vi "Main.vi"(11 "Module Admin":refnum<class "Delacor_lib_QMH_Module Admin.lvclass">) -> ()   [LabVIEW 2025, in "Keyboard.lvlib"]
doc: "60% keyboard. 0-9, a-z (lowercase and uppercase), and all the standard symbols."
uses:
  Keyboard.lvlib
  <vilib>/Delacor/Delacor QMH/Libraries/Module Admin_class/Delacor_lib_QMH_Module Admin.lvclass
  Module Data--cluster.ctl
  <vilib>/Delacor/Delacor QMH/Libraries/Message Queue_class/Delacor_lib_QMH_Message Queue.lvclass/Delacor_lib_QMH_Message Queue.ctl
  Stop Argument--cluster.ctl
  <vilib>/Delacor/Delacor QMH/Libraries/Module Admin_class/Delacor_lib_QMH_Module Admin.lvclass/Delacor_lib_QMH_Module Admin.ctl
  Get VI Refnum Argument--cluster.ctl
  Get VI Refnum (Reply Payload)--cluster.ctl
  <vilib>/Utility/miscctls.llb/LVPointTypeDef.ctl
  <vilib>/Delacor/Delacor QMH/Libraries/Module Admin_class/Delacor_lib_QMH_Get External Launch.vi
  <vilib>/Delacor/Delacor QMH/Libraries/Message Queue_class/Delacor_lib_QMH_Enqueue Message (Single).vi
  <vilib>/Delacor/Delacor QMH/Libraries/Message Queue_class/Delacor_lib_QMH_Message Queue.lvclass
panel:
  in  "Clear Buffer":bool
  in  "Tab":bool
  in  "Space":bool
  in  "Send":bool
  in  "Output Type":bool
  out "Buffer":string
  in  "=+":bool
  in  "-_":bool
  in  "\\|":bool
  in  "]}":bool
  in  "[{":bool
  in  "'\"":bool
  in  ";:":bool
  in  "/?":bool
  in  ".>":bool
  in  ",<":bool
  in  "Enter":bool
  in  "Backspace":bool
  in  "0)":bool
  in  "9(":bool
  in  "8*":bool
  in  "7&":bool
  in  "6^":bool
  in  "5%":bool
  in  "4$":bool
  in  "3#":bool
  in  "2@":bool
  in  "1!":bool
  in  "Shift Right":bool
  in  "Caps":bool
  in  "Shift Left":bool
  in  "zZ":bool
  in  "yY":bool
  in  "xX":bool
  in  "wW":bool
  in  "vV":bool
  in  "uU":bool
  in  "tT":bool
  in  "sS":bool
  in  "rR":bool
  in  "qQ":bool
  in  "pP":bool
  in  "oO":bool
  in  "nN":bool
  in  "mM":bool
  in  "lL":bool
  in  "kK":bool
  in  "jJ":bool
  in  "iI":bool
  in  "hH":bool
  in  "gG":bool
  in  "fF":bool
  in  "eE":bool
  in  "dD":bool
  in  "cC":bool
  in  "bB":bool
  in  "aA":bool
  out "error out":errorcluster
  out "Status":string
  in  "Simulate MHL Error":bool
  in  "Simulate EHL Error":bool
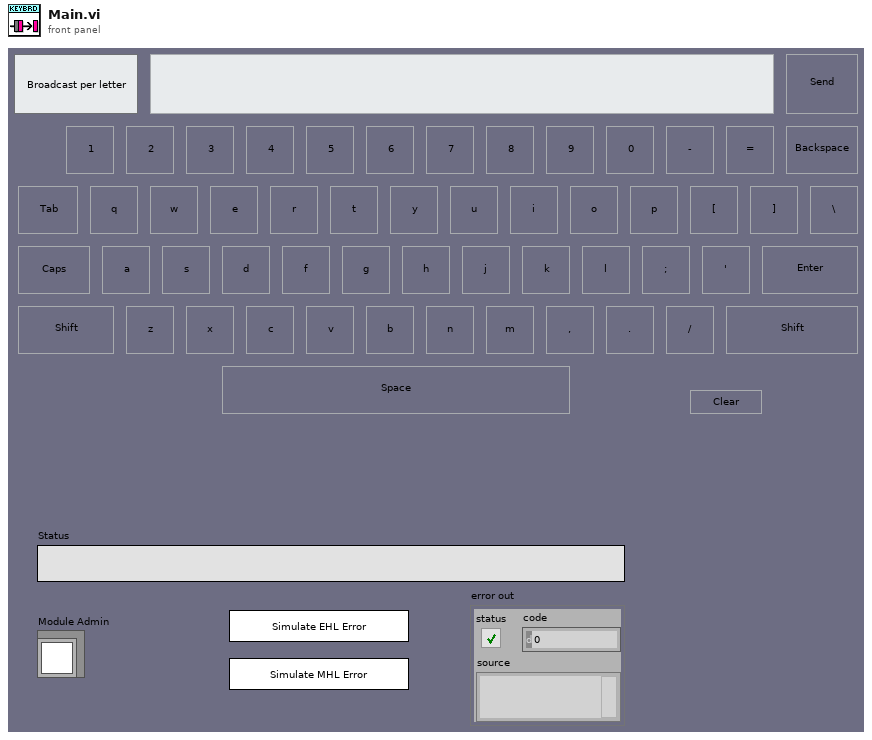
[diagram p1: front panel]
types:
  T1 = cluster{"=+":refnum<vi>, "-_":refnum<vi>, "\\|":refnum<vi>, "]}":refnum<vi>, "[{":refnum<vi>, "'\"":refnum<vi>, ";:":refnum<vi>, "/?":refnum<vi>, ".>":refnum<vi>, ",<":refnum<vi>, "0)":refnum<vi>, "9(":refnum<vi>, "8*":refnum<vi>, "7&":refnum<vi>, "6^":refnum<vi>, "5%":refnum<vi>, "4$":refnum<vi>, "3#":refnum<vi>, "2@":refnum<vi>, "1!":refnum<vi>, "eE":refnum<vi>, "rR":refnum<vi>, "cC":refnum<vi>, "kK":refnum<vi>, "yY":refnum<vi>, "fF":refnum<vi>, "gG":refnum<vi>, "hH":refnum<vi>, "mM":refnum<vi>, "zZ":refnum<vi>, "jJ":refnum<vi>, "uU":refnum<vi>, "tT":refnum<vi>, "sS":refnum<vi>, "wW":refnum<vi>, "xX":refnum<vi>, "iI":refnum<vi>, "qQ":refnum<vi>, "dD":refnum<vi>, "lL":refnum<vi>, "vV":refnum<vi>, "pP":refnum<vi>, "oO":refnum<vi>, "nN":refnum<vi>, "bB":refnum<vi>, "aA":refnum<vi>}
  T2 = typedef "Keyboard.lvlib/Request Events--cluster.ctl" = cluster{"Stop Module":refnum<user-event>, "Show Panel":refnum<user-event>, "Hide Panel":refnum<user-event>, "Get Module Execution Status":refnum<user-event>, "Show Diagram":refnum<user-event>, "Get VI Refnum":refnum<user-event>}
  T3 = typedef "Keyboard.lvlib/Module Data--cluster.ctl" = cluster{"Buffer":string, "Shift Status":bool}
  T4 = enum8{"Enabled", "Disabled", "Disabled and Grayed Out"}
  T5 = enum32{"invalid lock state", "Not Locked", "Locked (No Password)", "Password-protected"}
  T6 = typedef "Keyboard.lvlib/Stop Argument--cluster.ctl" = cluster{"Origin":string, "Exit via Stop Module Req?":bool, "Wait for Module to stop?":bool}
  T7 = typedef "Keyboard.lvlib/Get VI Refnum Argument--cluster.ctl" = cluster{"Wait Notifier":refnum<notifier>, "wait for reply":bool}
  T8 = typedef "LVPointTypeDef.ctl" = cluster{"Horizontal":i16, "Vertical":i16}
  T9 = enum32{"Invalid", "Standard", "Closed", "Hidden", "Minimized", "Maximized"}
  T10 = typedef "Keyboard.lvlib/Get VI Refnum (Reply Payload)--cluster.ctl" = cluster{"VI Refnum":refnum<vi>, "error":errorcluster}
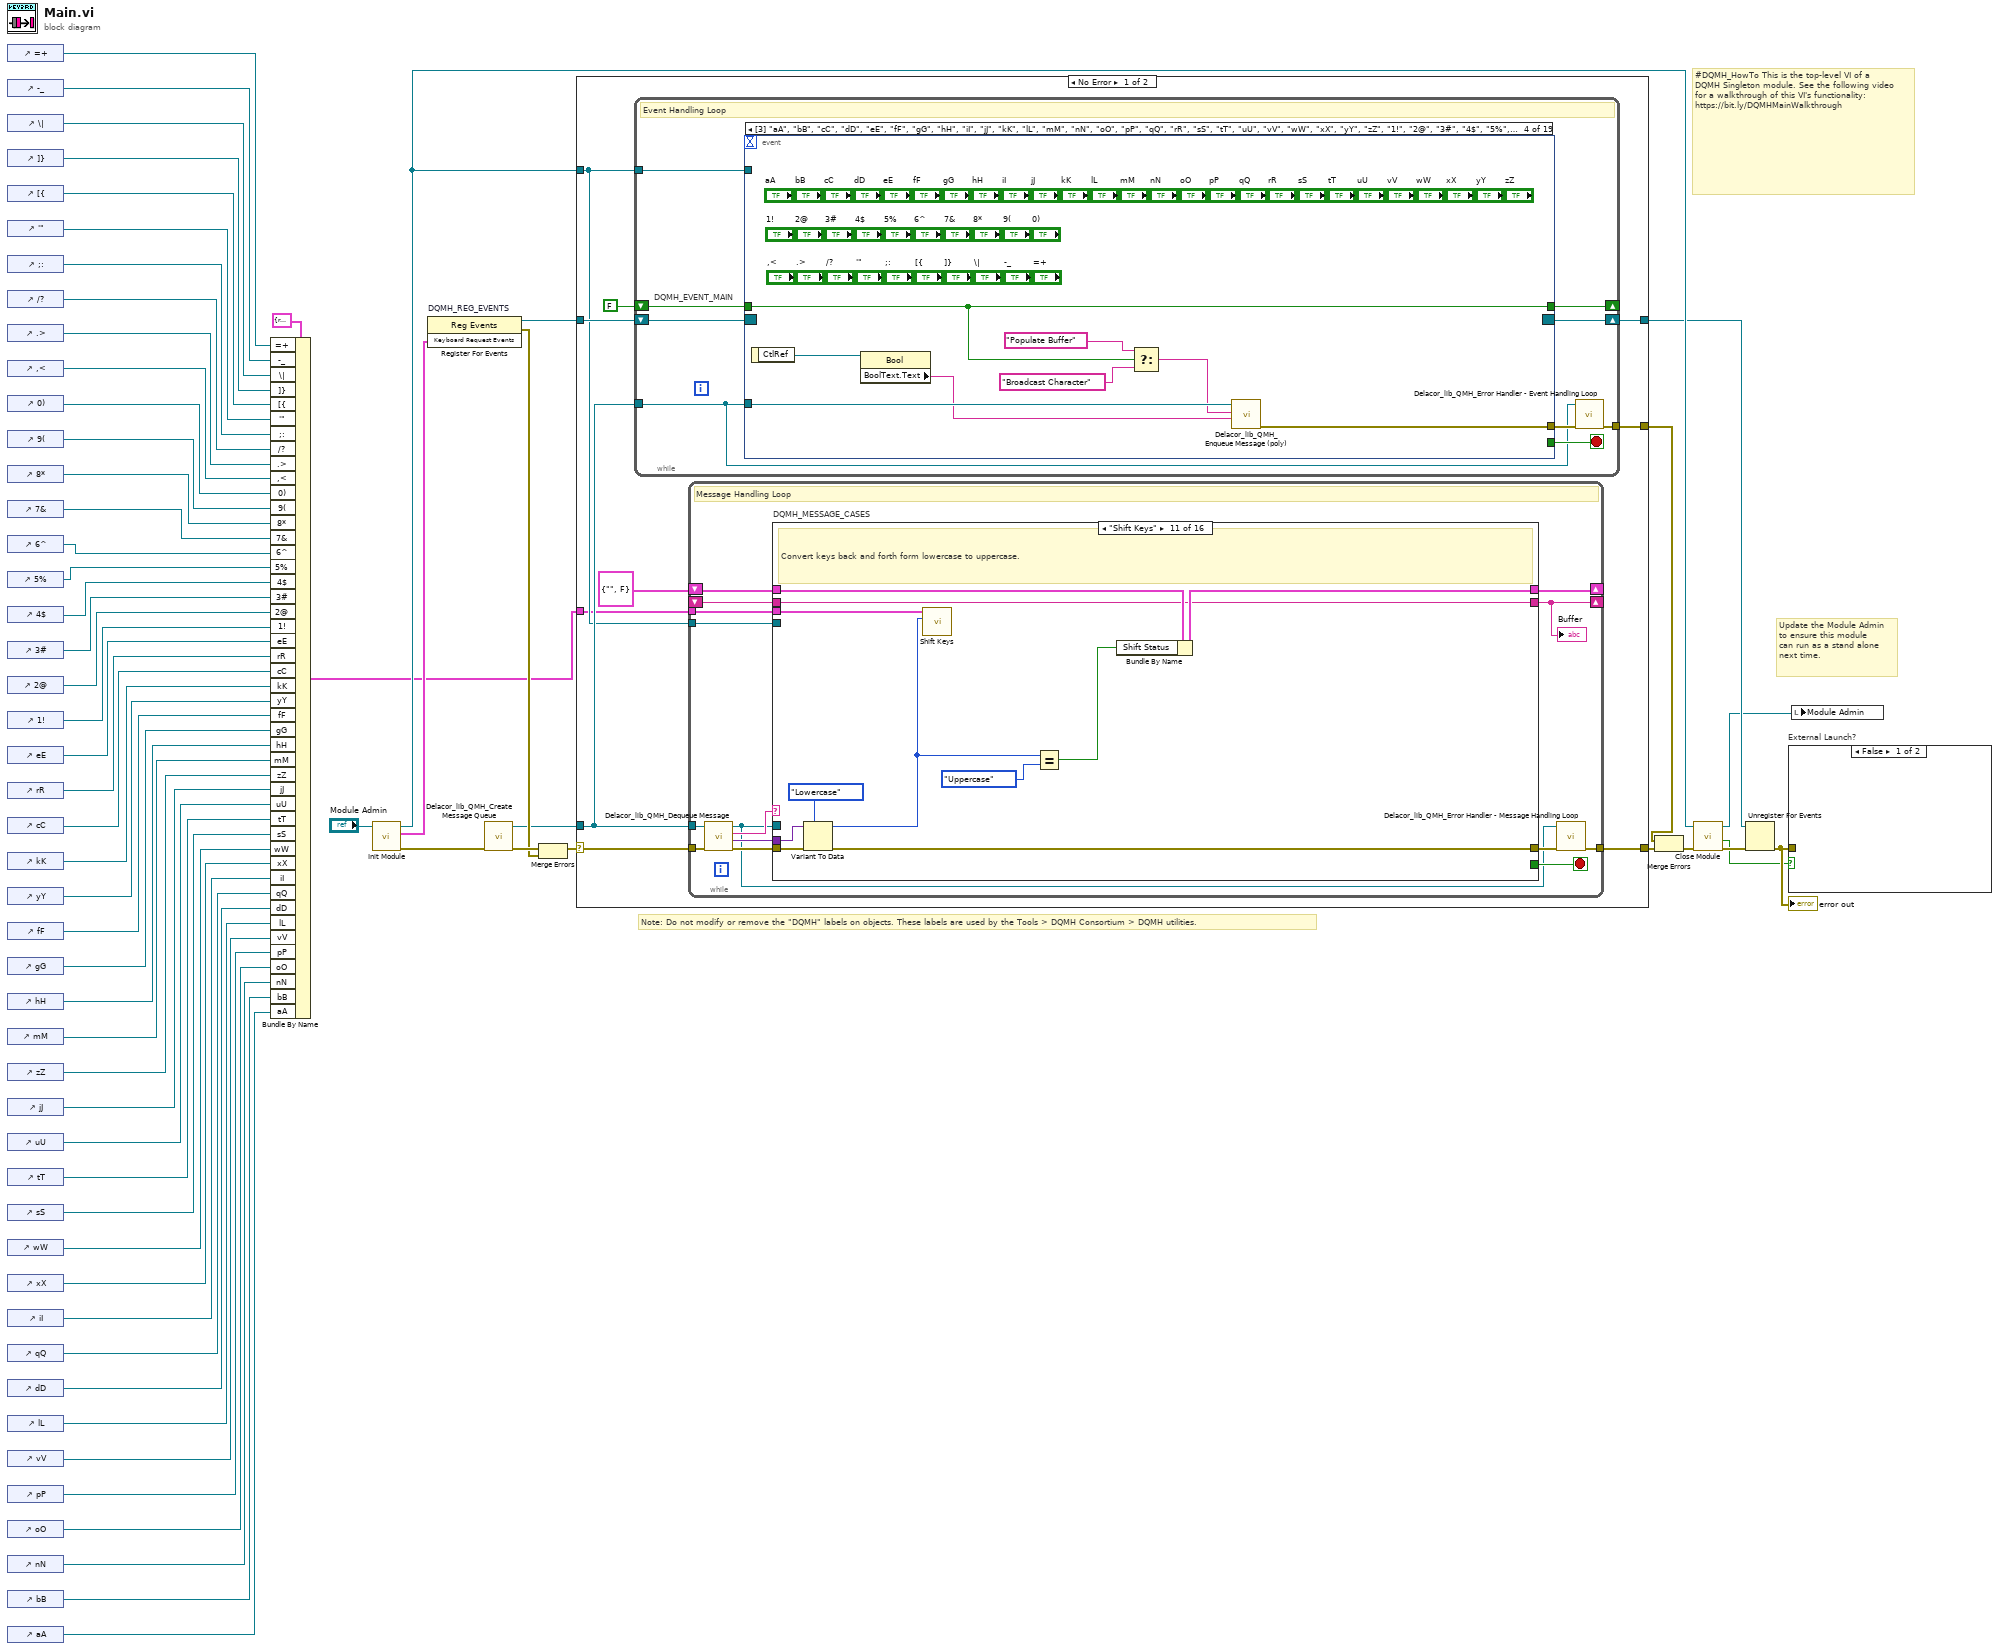
[diagram p0: block diagram]
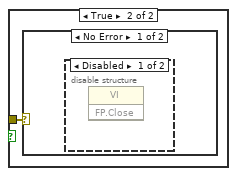
[diagram p2: hidden frame]
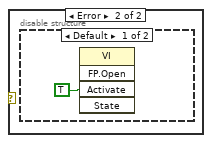
[diagram p4: hidden frame]
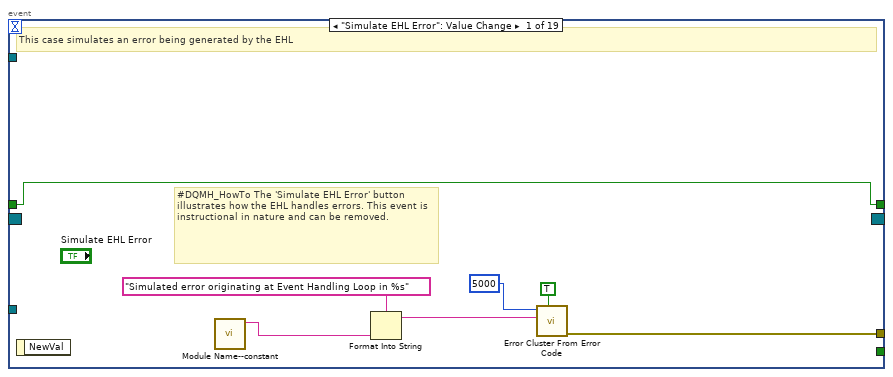
[diagram p6: hidden frame]
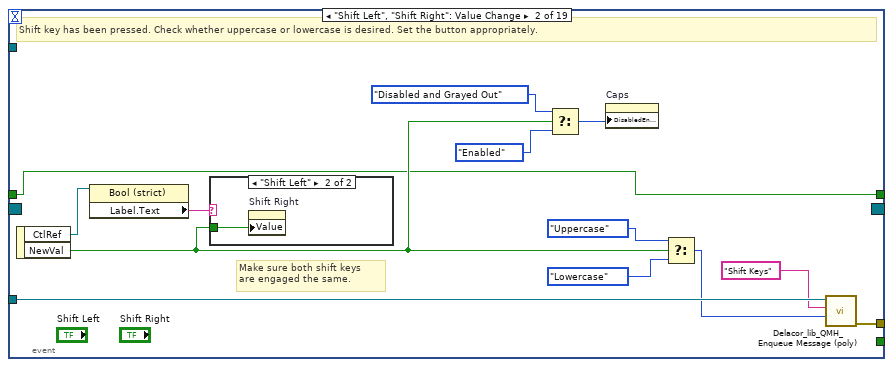
[diagram p7: hidden frame]
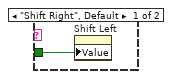
[diagram p8: hidden frame]
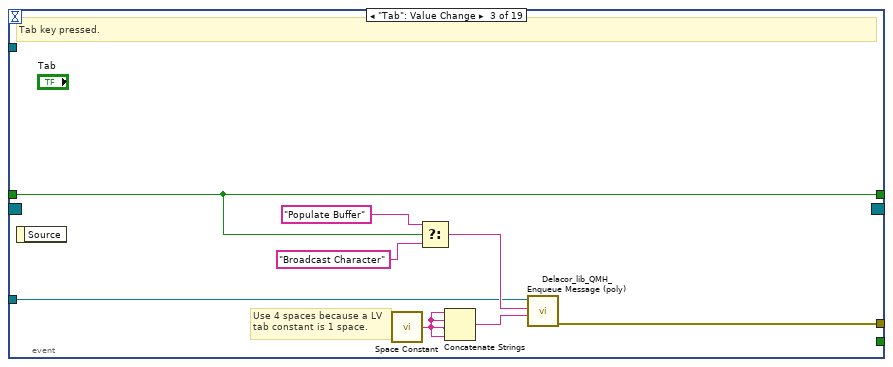
[diagram p9: hidden frame]
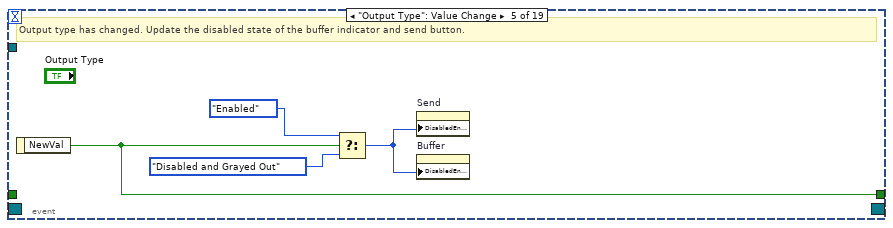
[diagram p10: hidden frame]
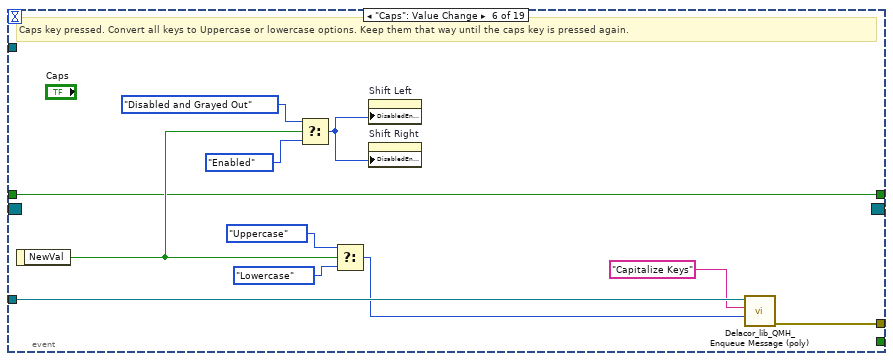
[diagram p11: hidden frame]
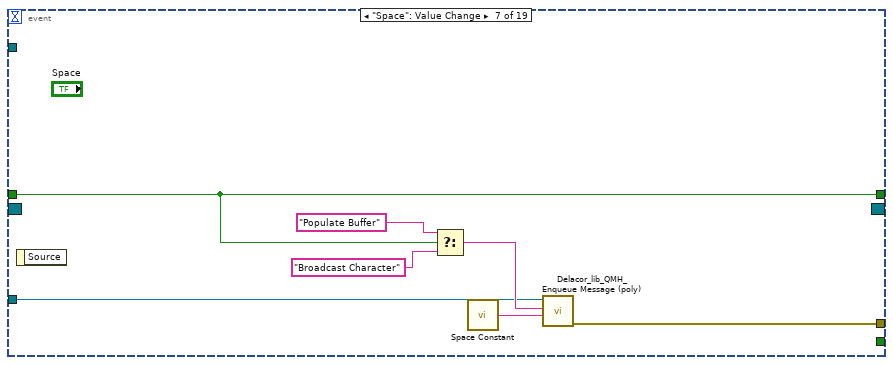
[diagram p12: hidden frame]
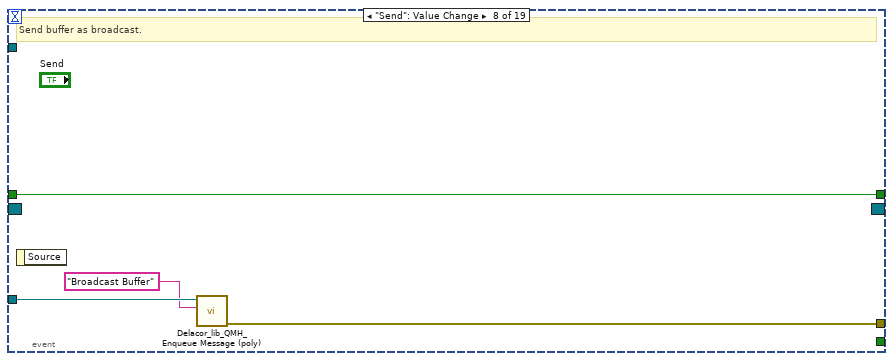
[diagram p13: hidden frame]
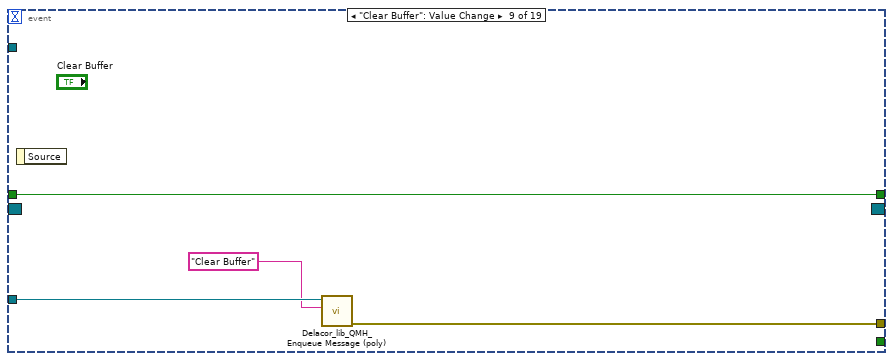
[diagram p14: hidden frame]
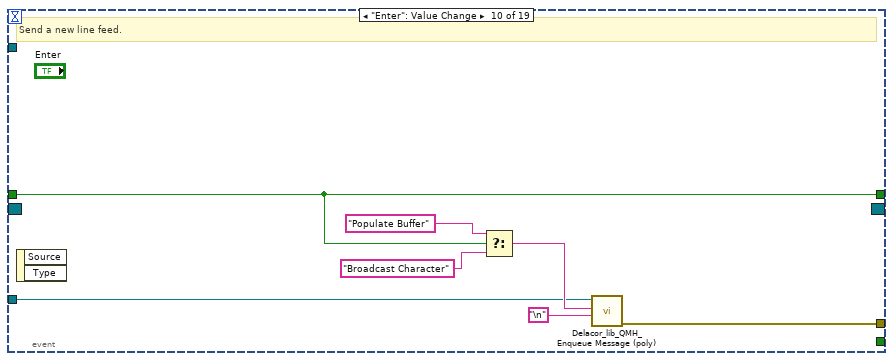
[diagram p15: hidden frame]
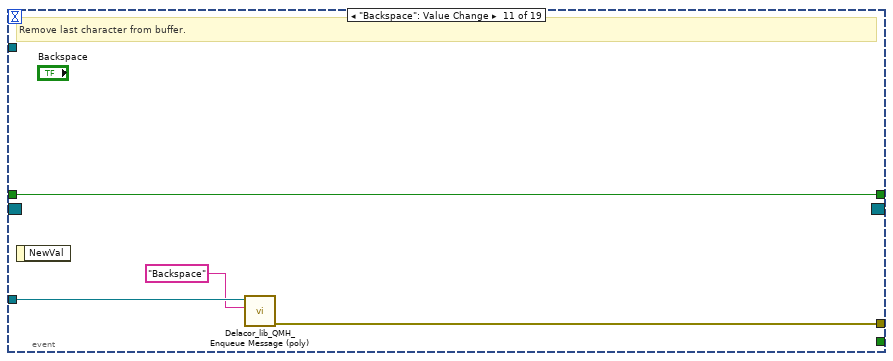
[diagram p16: hidden frame]
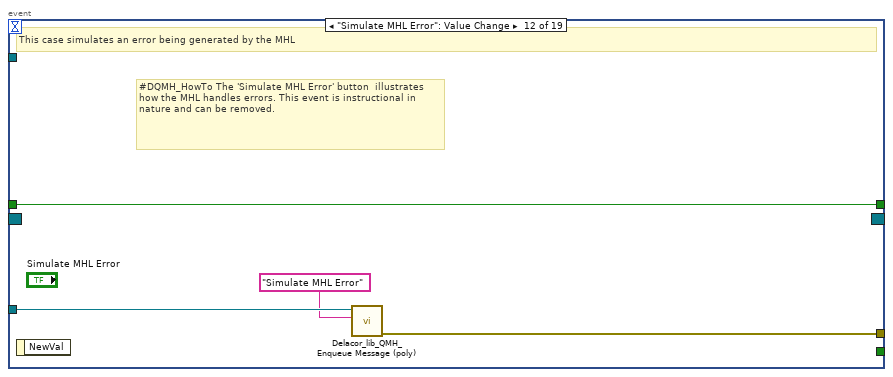
[diagram p17: hidden frame]
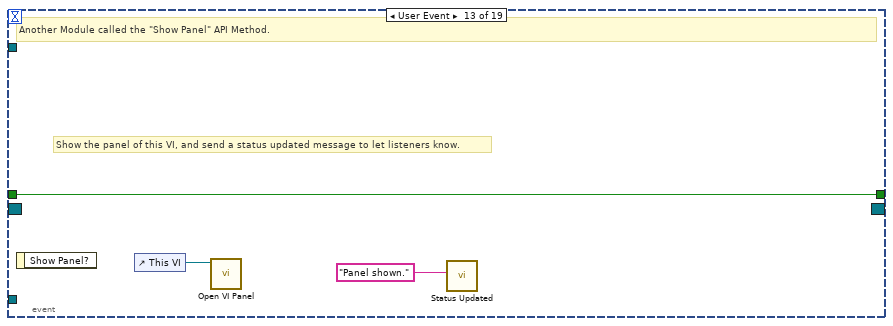
[diagram p18: hidden frame]
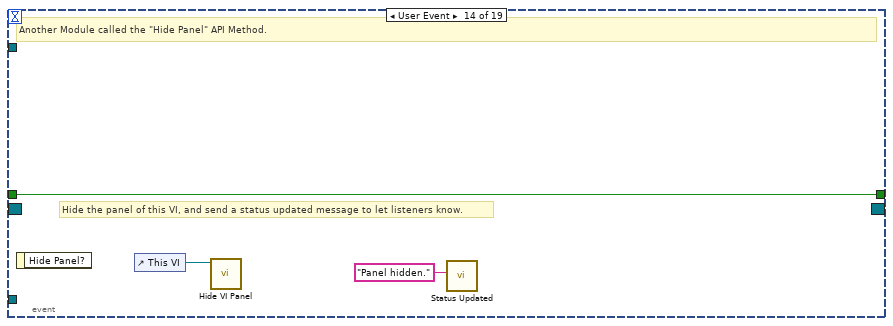
[diagram p19: hidden frame]
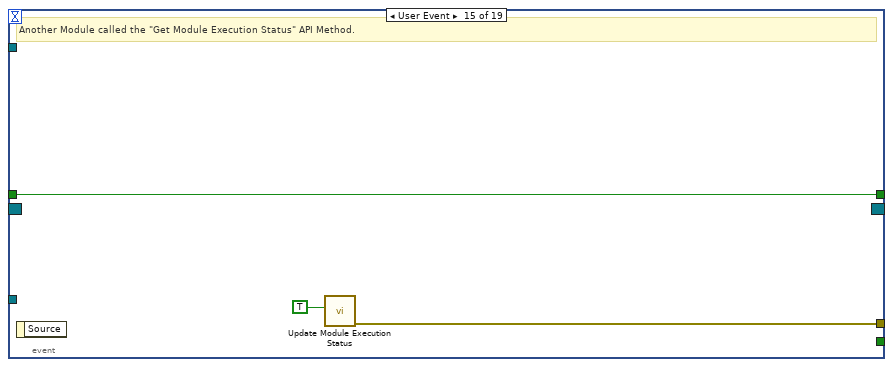
[diagram p20: hidden frame]
diagram:
  # "#DQMH_HowTo This is the top-level VI of a DQMH Singleton module. See the following video for a walkthrough of this VI's functionality: https://bit.ly/DQMHMainWalkthrough"
  # "Note: Do not modify or remove the \"DQMH\" labels on objects. These labels are used by the Tools > DQMH Consortium > DQMH utilities."
  # "Update the Module Admin to ensure this module can run as a stand alone next time."
  n1 = control-ref of="=+"() -> (w48:refnum<vi>)
  n2 = control-ref of="-_"() -> (w47:refnum<vi>)
  n3 = control-ref of="\\|"() -> (w46:refnum<vi>)
  n4 = control-ref of="]}"() -> (w45:refnum<vi>)
  n5 = control-ref of="[{"() -> (w44:refnum<vi>)
  n6 = control-ref of="'\""() -> (w43:refnum<vi>)
  n7 = control-ref of=";:"() -> (w42:refnum<vi>)
  n8 = control-ref of="/?"() -> (w41:refnum<vi>)
  n9 = control-ref of=".>"() -> (w40:refnum<vi>)
  n10 = control-ref of=",<"() -> (w39:refnum<vi>)
  n11 = control-ref of="0)"() -> (w38:refnum<vi>)
  n12 = control-ref of="9("() -> (w37:refnum<vi>)
  n13 = control-ref of="8*"() -> (w36:refnum<vi>)
  n14 = control-ref of="7&"() -> (w35:refnum<vi>)
  n15 = control-ref of="6^"() -> (w34:refnum<vi>)
  n16 = control-ref of="5%"() -> (w33:refnum<vi>)
  n17 = control-ref of="4$"() -> (w32:refnum<vi>)
  n18 = control-ref of="3#"() -> (w31:refnum<vi>)
  n19 = control-ref of="2@"() -> (w30:refnum<vi>)
  n20 = control-ref of="1!"() -> (w29:refnum<vi>)
  n21 = control-ref of="eE"() -> (w28:refnum<vi>)
  n22 = control-ref of="rR"() -> (w27:refnum<vi>)
  n23 = control-ref of="cC"() -> (w26:refnum<vi>)
  n24 = control-ref of="kK"() -> (w25:refnum<vi>)
  n25 = control-ref of="yY"() -> (w24:refnum<vi>)
  n26 = control-ref of="fF"() -> (w23:refnum<vi>)
  n27 = control-ref of="gG"() -> (w22:refnum<vi>)
  n28 = control-ref of="hH"() -> (w21:refnum<vi>)
  n29 = control-ref of="mM"() -> (w20:refnum<vi>)
  n30 = control-ref of="zZ"() -> (w19:refnum<vi>)
  n31 = control-ref of="jJ"() -> (w18:refnum<vi>)
  n32 = control-ref of="uU"() -> (w17:refnum<vi>)
  n33 = control-ref of="tT"() -> (w16:refnum<vi>)
  n34 = control-ref of="sS"() -> (w15:refnum<vi>)
  n35 = control-ref of="wW"() -> (w14:refnum<vi>)
  n36 = control-ref of="xX"() -> (w13:refnum<vi>)
  n37 = control-ref of="iI"() -> (w12:refnum<vi>)
  n38 = control-ref of="qQ"() -> (w11:refnum<vi>)
  n39 = control-ref of="dD"() -> (w10:refnum<vi>)
  n40 = control-ref of="lL"() -> (w9:refnum<vi>)
  n41 = control-ref of="vV"() -> (w8:refnum<vi>)
  n42 = control-ref of="pP"() -> (w7:refnum<vi>)
  n43 = control-ref of="oO"() -> (w6:refnum<vi>)
  n44 = control-ref of="nN"() -> (w5:refnum<vi>)
  n45 = control-ref of="bB"() -> (w4:refnum<vi>)
  n46 = control-ref of="aA"() -> (w3:refnum<vi>)
  n47 = Bundle By Name(cluster=T1 {"=+"=refnum, "-_"=refnum, "\\|"=refnum, "]}"=refnum, "[{"=refnum, "'\""=refnum, ";:"=refnum, "/?"=refnum, ".>"=refnum, ",<"=refnum, "0)"=refnum, "9("=refnum, "8*"=refnum, "7&"=refnum, "6^"=refnum, "5%"=refnum, "4$"=refnum, "3#"=refnum, "2@"=refnum, "1!"=refnum, "eE"=refnum, "rR"=refnum, "cC"=refnum, "kK"=refnum, "yY"=refnum, "fF"=refnum, "gG"=refnum, "hH"=refnum, "mM"=refnum, "zZ"=refnum, "jJ"=refnum, "uU"=refnum, "tT"=refnum, "sS"=refnum, "wW"=refnum, "xX"=refnum, "iI"=refnum, "qQ"=refnum, "dD"=refnum, "lL"=refnum, "vV"=refnum, "pP"=refnum, "oO"=refnum, "nN"=refnum, "bB"=refnum, "aA"=refnum}, "=+"=w48, "-_"=w47, "\\|"=w46, "]}"=w45, "[{"=w44, "'\""=w43, ";:"=w42, "/?"=w41, ".>"=w40, ",<"=w39, "0)"=w38, "9("=w37, "8*"=w36, "7&"=w35, "6^"=w34, "5%"=w33, "4$"=w32, "3#"=w31, "2@"=w30, "1!"=w29, "eE"=w28, "rR"=w27, "cC"=w26, "kK"=w25, "yY"=w24, "fF"=w23, "gG"=w22, "hH"=w21, "mM"=w20, "zZ"=w19, "jJ"=w18, "uU"=w17, "tT"=w16, "sS"=w15, "wW"=w14, "xX"=w13, "iI"=w12, "qQ"=w11, "dD"=w10, "lL"=w9, "vV"=w8, "pP"=w7, "oO"=w6, "nN"=w5, "bB"=w4, "aA"=w3) -> (w1:T1)
  n48 = call "Init Module.vi"("Singleton Module Admin in"="Module Admin") -> ("error out"=w64:errorcluster, "Keyboard Request Events"=w53:T2, "Singleton Module Admin out"=w56:refnum<class "Delacor_lib_QMH_Module Admin.lvclass">)  [unwired: 8 in]
  n49 = register-events "DQMH_REG_EVENTS"(w53) -> (reference out=w54:refnum<event-registration>, error out=w57:errorcluster)  [unwired: 2 in]
  n50 = call <vilib>:"Delacor_lib_QMH_Create Message Queue.vi"("error in"=w64) -> ("error out"=w59:errorcluster, "Message Queue"=w52:refnum<class "Delacor_lib_QMH_Message Queue.lvclass">)  [unwired: 9 in]
  n51 = Merge Errors(w59, w57) -> (w58:errorcluster)
  n52 = case shown="No Error" w58 {
    selector: w58 -> [w73 w406]
    tunnel: [w75 w405] -> w65
    tunnel: [w72 w404] -> w55
    tunnel: w54 -> [w70 w404]
    tunnel: w52 -> [w69 w399]
    tunnel: [w74 _] -> w62
    tunnel: w56 -> [w68 w400]
    tunnel: w1 -> [w67 _]
    frame No Error {
      n53 = while {
        tunnel: w69 -> [w78]
        shift-right: [w81] -> w72
        shift-left: w70 -> [w82]
        tunnel: [w83] -> w74
        tunnel: w68 -> [w79]
        shift-right: [w77] -> _
        shift-left: FALSE ("NewVal") -> [w76]
        stop <- w80 stop-if-true
        # "Event Handling Loop"
        n54 = event "DQMH_EVENT_MAIN" shown="[3] \"aA\", \"bB\", \"cC\", \"dD\", \"eE\", \"fF\", \"gG\", \"hH\", \"iI\", \"jJ\", \"kK\", \"lL\", \"mM\", \"nN\", \"oO\", \"pP\", \"qQ\", \"rR\", \"sS\", \"tT\", \"uU\", \"vV\", \"wW\", \"xX\", \"yY\", \"zZ\", \"1!\", \"2@\", \"3#\", \"4$\", \"5%\", \"6^\", \"7&\", \"8*\", \"9(\", \"0)\", \",<\", \".>\", \"/?\", \";:\", \"'\"\", \"[{\", \"]}\", \"\\|\", \"-_\", \"=+\": Value Change" {
          selector: w82 -> [_ _ _ _ _ _ _ _ _ _ _ _ _ _ _ _ _ _ _]
          dyn-events: [_ _ _ _ _ _ _ _ _ _ _ _ _ _ _ _ _ _ _] -> w81
          timeout: _ -> [_ _ _ _ _ _ _ _ _ _ _ _ _ _ _ _ _ _ _]
          tunnel: [_ _ _ _ _ _ _ _ _ _ _ _ _ _ _ _ TRUE ("Discard?") _ _] -> w80
          tunnel: w78 -> [_ w104 w110 w121 _ w137 w141 w148 w152 w154 w163 w166 _ _ _ _ w195 w203 w219]
          tunnel: [w91 w103 w109 w120 _ w136 w140 w147 w151 w153 w162 w167 _ _ w176 _ w198 w205 w213] -> w84
          tunnel: w79 -> [_ _ _ _ _ _ _ _ _ _ _ _ _ _ _ _ _ w202 _]
          tunnel: [w85 w92 w107 w115 w123 w127 w139 w145 w149 w156 w160 w164 w168 w171 w174 w177 w187 w200 w220] -> w77
          tunnel: w76 -> [w85 w92 w107 w115 _ w127 w139 w145 w149 w156 w160 w164 w168 w171 w174 w177 w187 w200 w220]
          event "Simulate EHL Error": Value Change {
            # "#DQMH_HowTo The 'Simulate EHL Error' button  illustrates how the EHL handles errors. This event is instructional in nature and can be removed."
            # "This case simulates an error being generated by the EHL"
            n55 = event-data() -> ()  [unwired: 1 in, 1 out]
            n56 = call "Module Name--constant.vi"() -> ("Module Name"=w88:string)  [unwired: 11 in]
            n57 = Format Into String(format string="Simulated error originating at Event Handling Loop in %s", w88) -> (resulting string=w89:string)  [unwired: 2 in, 1 out]
            n58 = call <vilib>:"Error Cluster From Error Code.vi"("show call chain? (False)"=TRUE, "error message (\"\")"=w89, "error code (0)"=5000) -> ("error out"=w91:errorcluster)  [unwired: 6 in]
          }
          event "Shift Left", "Shift Right": Value Change {
            # "Make sure both shift keys\nare engaged the same."
            # "Shift key has been pressed. Check whether uppercase or lowercase is desired. Set the button appropriately."
            n59 = event-data() -> ("CtlRef"=w98:refnum<vi>, "NewVal"=w94:bool)  [unwired: 1 in]
            n60 = property class="Bool (strict)"(reference=w98) -> ("Label.Text"=w97:string)  [unwired: 1 in, 2 out]
            n61 = case shown="\"Shift Left\"" w97 {
              tunnel: w94 -> [w105 w106]
              frame "Shift Right", Default {
                n62 = property on="Shift Left" class="Bool (strict)"("Value"=w105) -> ()  [unwired: 2 in, 2 out]
              }
              frame "Shift Left" {
                n63 = property on="Shift Right" class="Bool (strict)"("Value"=w106) -> ()  [unwired: 2 in, 2 out]
              }
            }
            n64 = Select(t=T4."Disabled and Grayed Out" ("Disabled"), s=w94, f=T4."Enabled" ("Disabled")) -> (s? t:f=w93:T4)
            n65 = property on="Caps" class="Bool (strict)"("DisabledEnum"=w93) -> ()  [unwired: 2 in, 2 out]
            n66 = Select(t=enum16{"Uppercase", "Lowercase"}."Uppercase" ("Upper / Lower Case"), s=w94, f=enum16{"Uppercase", "Lowercase"}."Lowercase" ("Upper / Lower Case")) -> (s? t:f=w99:enum16{"Uppercase", "Lowercase"})
            n67 = call-poly <vilib>:"Delacor_lib_QMH_Enqueue Message (poly).vi"("Message Data"=w99, "Message"="Shift Keys", "Message Queue in"=w104) -> ("error out"=w103:errorcluster)  [unwired: 7 in, 1 out]
          }
          event "Tab": Value Change {
            # "Use 4 spaces because a LV\ntab constant is 1 space."
            # "Tab key pressed."
            n68 = event-data() -> ()  [unwired: 1 in, 1 out]
            n69 = call <vilib>:"Space Constant.vi"() -> ("String"=w114:string)
            n70 = Select(t="Populate Buffer", s=w107, f="Broadcast Character" ("t")) -> (s? t:f=w113:string)
            n71 = Concatenate Strings(w114, w114, w114, w114) -> (w108:string)
            n72 = call-poly <vilib>:"Delacor_lib_QMH_Enqueue Message (poly).vi"("Message Data"=w108, "Message"=w113, "Message Queue in"=w110) -> ("error out"=w109:errorcluster)  [unwired: 7 in, 1 out]
          }
          event "aA", "bB", "cC", "dD", "eE", "fF", "gG", "hH", "iI", "jJ", "kK", "lL", "mM", "nN", "oO", "pP", "qQ", "rR", "sS", "tT", "uU", "vV", "wW", "xX", "yY", "zZ", "1!", "2@", "3#", "4$", "5%", "6^", "7&", "8*", "9(", "0)", ",<", ".>", "/?", ";:", "'\"", "[{", "]}", "\\|", "-_", "=+": Value Change {
            n73 = event-data() -> ("CtlRef"=w122:refnum<vi>)  [unwired: 1 in]
            n74 = property class="Bool"(reference=w122) -> ("BoolText.Text"=w118:string)  [unwired: 1 in, 2 out]
            n75 = Select(t="Populate Buffer", s=w115, f="Broadcast Character" ("t")) -> (s? t:f=w119:string)
            n76 = call-poly <vilib>:"Delacor_lib_QMH_Enqueue Message (poly).vi"("Message Data"=w118, "Message"=w119, "Message Queue in"=w121) -> ("error out"=w120:errorcluster)  [unwired: 7 in, 1 out]
          }
          event "Output Type": Value Change {
            # "Output type has changed. Update the disabled state of the buffer indicator and send button."
            n77 = event-data() -> ("NewVal"=w123:bool)  [unwired: 1 in]
            n78 = Select(t=T4."Enabled" ("Disabled"), s=w123, f=T4."Disabled and Grayed Out" ("Disabled")) -> (s? t:f=w125:T4)
            n79 = property on="Send" class="Bool"("DisabledEnum"=w125) -> ()  [unwired: 2 in, 2 out]
            n80 = property on="Buffer" class="Str"("DisabledEnum"=w125) -> ()  [unwired: 2 in, 2 out]
          }
          event "Caps": Value Change {
            # "Caps key pressed. Convert all keys to Uppercase or lowercase options. Keep them that way until the caps key is pressed again."
            n81 = event-data() -> ("NewVal"=w131:bool)  [unwired: 1 in]
            n82 = Select(t=T4."Disabled and Grayed Out" ("Disabled"), s=w131, f=T4."Enabled" ("Disabled")) -> (s? t:f=w128:T4)
            n83 = Select(t=enum16{"Uppercase", "Lowercase"}."Uppercase" ("Upper / Lower Case"), s=w131, f=enum16{"Uppercase", "Lowercase"}."Lowercase" ("Upper / Lower Case")) -> (s? t:f=w132:enum16{"Uppercase", "Lowercase"})
            n84 = property on="Shift Left" class="Bool (strict)"("DisabledEnum"=w128) -> ()  [unwired: 2 in, 2 out]
            n85 = property on="Shift Right" class="Bool (strict)"("DisabledEnum"=w128) -> ()  [unwired: 2 in, 2 out]
            n86 = call-poly <vilib>:"Delacor_lib_QMH_Enqueue Message (poly).vi"("Message Data"=w132, "Message"="Capitalize Keys", "Message Queue in"=w137) -> ("error out"=w136:errorcluster)  [unwired: 7 in, 1 out]
          }
          event "Space": Value Change {
            n87 = event-data() -> ()  [unwired: 1 in, 1 out]
            n88 = Select(t="Populate Buffer", s=w139, f="Broadcast Character" ("t")) -> (s? t:f=w144:string)
            n89 = call <vilib>:"Space Constant.vi"() -> ("String"=w138:string)
            n90 = call-poly <vilib>:"Delacor_lib_QMH_Enqueue Message (poly).vi"("Message Data"=w138, "Message"=w144, "Message Queue in"=w141) -> ("error out"=w140:errorcluster)  [unwired: 7 in, 1 out]
          }
          event "Send": Value Change {
            # "Send buffer as broadcast."
            n91 = event-data() -> ()  [unwired: 1 in, 1 out]
            n92 = call-poly <vilib>:"Delacor_lib_QMH_Enqueue Message (poly).vi"("Message"="Broadcast Buffer", "Message Queue in"=w148) -> ("error out"=w147:errorcluster)  [unwired: 8 in, 1 out]
          }
          event "Clear Buffer": Value Change {
            n93 = event-data() -> ()  [unwired: 1 in, 1 out]
            n94 = call-poly <vilib>:"Delacor_lib_QMH_Enqueue Message (poly).vi"("Message"="Clear Buffer", "Message Queue in"=w152) -> ("error out"=w151:errorcluster)  [unwired: 8 in, 1 out]
          }
          event "Enter": Value Change {
            # "Send a new line feed."
            n95 = event-data() -> ()  [unwired: 1 in, 2 out]
            n96 = Select(t="Populate Buffer", s=w156, f="Broadcast Character" ("t")) -> (s? t:f=w159:string)
            n97 = call-poly <vilib>:"Delacor_lib_QMH_Enqueue Message (poly).vi"("Message Data"="\n", "Message"=w159, "Message Queue in"=w154) -> ("error out"=w153:errorcluster)  [unwired: 7 in, 1 out]
          }
          event "Backspace": Value Change {
            # "Remove last character from buffer."
            n98 = event-data() -> ()  [unwired: 1 in, 1 out]
            n99 = call-poly <vilib>:"Delacor_lib_QMH_Enqueue Message (poly).vi"("Message"="Backspace", "Message Queue in"=w163) -> ("error out"=w162:errorcluster)  [unwired: 8 in, 1 out]
          }
          event "Simulate MHL Error": Value Change {
            # "#DQMH_HowTo The 'Simulate MHL Error' button  illustrates how the MHL handles errors. This event is instructional in nature and can be removed."
            # "This case simulates an error being generated by the MHL"
            n100 = event-data() -> ()  [unwired: 1 in, 1 out]
            n101 = call-poly <vilib>:"Delacor_lib_QMH_Enqueue Message (poly).vi"("Message"="Simulate MHL Error", "Message Queue in"=w166) -> ("error out"=w167:errorcluster)  [unwired: 8 in, 1 out]
          }
          event User Event {
            # "Show the panel of this VI, and send a status updated message to let listeners know."
            # "Another Module called the \"Show Panel\" API Method."
            n102 = event-data() -> ()  [unwired: 1 in, 1 out]
            n103 = control-ref of="This VI"() -> (w170:refnum<vi>)
            n104 = call "Open VI Panel.vi"("VI"=w170) -> ()  [unwired: 10 in, 1 out]
            n105 = call "Status Updated.vi"("Status"="Panel shown." ("format string")) -> ()  [unwired: 10 in, 1 out]
          }
          event User Event {
            # "Hide the panel of this VI, and send a status updated message to let listeners know."
            # "Another Module called the \"Hide Panel\" API Method."
            n106 = event-data() -> ()  [unwired: 1 in, 1 out]
            n107 = control-ref of="This VI"() -> (w173:refnum<vi>)
            n108 = call "Hide VI Panel.vi"("VI"=w173) -> ()  [unwired: 10 in, 1 out]
            n109 = call "Status Updated.vi"("Status"="Panel hidden." ("format string")) -> ()  [unwired: 10 in, 1 out]
          }
          event User Event {
            # "Another Module called the \"Get Module Execution Status\" API Method."
            n110 = event-data() -> ()  [unwired: 1 in, 1 out]
            n111 = call "Update Module Execution Status.vi"("Running?"=TRUE) -> ("error out"=w176:errorcluster)  [unwired: 10 in]
          }
          event User Event {
            # "Another Module called the \"Show Diagram\" API Method. This event is used for debugging."
            n112 = event-data() -> ()  [unwired: 1 in, 1 out]
            n113 = disable-structure shown="RUN_TIME_ENGINE==False" {
              frame condition #0 (active) {
                # "functionality not available in exe"
                n114 = invoke on="Invoke Node" class="VI" method="Lock State.Get"() -> (error out=w183:errorcluster, "Get Lock State"=w182:T5, "pwd in cache"=w179:bool)  [unwired: 4 in, 1 out]
                n115 = Equal?(x=T5."Password-protected", y=w182) -> (x = y?=w180:bool)
                n116 = Compound Arithmetic op=AND(w180, invert w179) -> (w178:bool)
                n117 = case shown="False" w178 {
                  tunnel: w183 -> [w186 _]
                  frame False {
                    n118 = property on="Property Node" class="VI"(error in=w186, "BDWin.Open"=TRUE ("Block Diagram Window:Open")) -> ()  [unwired: 1 in, 2 out]
                    n119 = call "Status Updated.vi"("Status"="Block Diagram shown." ("format string")) -> ()  [unwired: 10 in, 1 out]
                  }
                  frame True {
                    # "Password-protected VI, and the password is not in the cache. Do not show the diagram."
                  }
                }
              }
              frame condition #1 {
              }
            }
          }
          event User Event {
            # "The Stop Module Event can get fired from the Exit message in the MHL. The queue gets destroyed in that case. If the queue no longer exists, the Enqueue Exit as a priority message will return error 1. It is safe to ignore, because the module is already exiting."
            # "Another Module called the \"Stop Module\" API Method  or the Message Handling Loop below."
            n120 = event-data() -> ("Origin"=w194:string, "Exit via Stop Module Req?"=w190:bool, "Wait for Module to stop?"=w189:bool)  [unwired: 1 in]
            n121 = local write "Status"(w194) -> ()
            n122 = Bundle By Name(cluster=T6 {"Origin"="", "Exit via Stop Module Req?"=FALSE, "Wait for Module to stop?"=FALSE} ("Stop Argument"), "Exit via Stop Module Req?"=w190, "Wait for Module to stop?"=w189) -> (w188:T6)
            n123 = call-poly <vilib>:"Delacor_lib_QMH_Enqueue Message (poly).vi"("Priority Message? (F)"=TRUE, "Message Data"=w188, "Message"="Exit", "Message Queue in"=w195) -> ("error out"=w199:errorcluster)  [unwired: 6 in, 1 out]
            n124 = call <vilib>:"Clear Errors.vi"("error in (no error)"=w199, "specific error code to clear (0: all)"=1) -> ("error out"=w198:errorcluster)  [unwired: 4 in, 1 out]
          }
          event Panel Close? {
            w204 = TRUE  # Discard the event, the MHL is responsible for closing and stopping this VI.
            # "Hide the panel or send the 'Exit' message if the user clicks the 'X' on the module main VI panel."
            n125 = event-data() -> ()  [unwired: 1 in, 1 out]
            n126 = property on="Property Node" class="Module Admin"(reference=w202) -> ("Accessors:External Launch"=w201:bool)  [unwired: 1 in, 2 out]
            n127 = case shown="False" w201 {
              tunnel: w203 -> [_ w211]
              tunnel: [_ w212] -> w205
              frame True {
                # "If externally launched, clicking the 'X' hides the panel, but doesn't close it."
                n128 = control-ref of="This VI"() -> (w208:refnum<vi>)
                n129 = call "Hide VI Panel.vi"("VI"=w208) -> ("error out"=w206:errorcluster)  [unwired: 10 in]
                n130 = call "Status Updated.vi"("error in"=w206, "Status"="Panel hidden." ("format string")) -> ()  [unwired: 9 in, 1 out]
              }
              frame False {
                # "If run as a stand-alone VI, clicking the panel 'X' stops the VI."
                n131 = call-poly <vilib>:"Delacor_lib_QMH_Enqueue Message (poly).vi"("Priority Message? (F)"=TRUE, "Message"="Exit", "Message Queue in"=w211) -> ("error out"=w212:errorcluster)  [unwired: 7 in, 1 out]
              }
            }
            n132 = event-data ("Event Filter Node")("Discard?"=w204) -> ()  [unwired: 1 in, 1 out]
          }
          event User Event {
            # "Another Module called the \"Get VI Refnum\" API Method."
            n133 = event-data() -> ("Wait Notifier"=w215:refnum<notifier>, "wait for reply"=w214:bool)  [unwired: 1 in]
            n134 = Bundle(cluster=T7 {"Wait Notifier"=refnum, "wait for reply"=FALSE} ("Get VI Refnum Argument"), "Wait Notifier"=w215, "wait for reply"=w214) -> (w216:T7)
            n135 = call-poly <vilib>:"Delacor_lib_QMH_Enqueue Message (poly).vi"("Message Data"=w216, "Message"="Get VI Refnum", "Message Queue in"=w219) -> ("error out"=w213:errorcluster)  [unwired: 7 in, 1 out]
          }
        }
        n136 = call-dynamic "Delacor_lib_QMH_Error Handler - Event Handling Loop.vi"("error in"=w84, "Message Queue in"=w78) -> ("dup error in"=w83:errorcluster)  [unwired: 8 in, 1 out]
      }
      n137 = while {
        tunnel: w69 -> [w224]
        shift-right: [w232] -> _
        shift-left: T3 {"Buffer"="", "Shift Status"=FALSE} ("Data Cluster") -> [w233]
        tunnel: w73 -> [w235]
        tunnel: [w227] -> w75
        tunnel: w68 -> [w228]
        tunnel: w67 -> [w223]
        shift-right: [w222] -> _
        shift-left: _ -> [w221]
        stop <- w231 stop-if-true
        # "Message Handling Loop"
        n138 = call-dynamic "Delacor_lib_QMH_Dequeue Message.vi"("error in"=w235, "Message Queue in"=w224) -> ("error out"=w234:errorcluster, "Message Data"=w229:variant, "Message"=w230:string, "Message Queue out"=w225:refnum<class "Delacor_lib_QMH_Message Queue.lvclass">)  [unwired: 6 in]
        n139 = case "DQMH_MESSAGE_CASES" shown="\"Shift Keys\"" w230 {
          selector: w230 -> [_ _ _ _ _ _ _ _ _ _ _ _ _ _ _ w394]
          tunnel: w225 -> [_ _ _ _ _ _ _ _ _ _ _ _ _ w358 w381 _]
          tunnel: w234 -> [w257 w262 w275 w281 w285 w290 w294 w307 w317 w329 w340 w343 w353 w365 w387 w397]
          tunnel: [w255 w262 w264 w280 w285 w288 w294 w303 w316 w326 w337 w343 w352 w361 w382 w398] -> w226
          tunnel: w233 -> [w246 w261 w274 w279 w284 w287 w293 w300 w313 w328 w339 w342 w350 w360 w380 w395]
          tunnel: [w245 w261 w274 w279 w283 w287 w292 w300 w311 w328 w332 w342 w350 w360 w380 w395] -> w232
          tunnel: [_ _ _ _ _ _ _ _ _ _ _ _ _ _ w379 _] -> w231
          tunnel: w229 -> [_ _ w271 _ _ _ _ w306 w315 w325 w336 _ _ w359 w378 _]
          tunnel: w228 -> [w247 _ _ _ _ _ _ _ _ _ _ _ _ w357 w373 _]
          tunnel: w223 -> [_ _ _ _ _ _ _ _ _ w327 w338 _ _ _ _ _]
          tunnel: [w237 w260 w273 w278 w282 w289 w291 w301 w309 w322 w330 w341 w344 w354 w372 w388] -> w222
          tunnel: w221 -> [_ w260 w273 w278 _ w289 _ w301 _ w322 w330 w341 w344 w354 w372 w388]
          frame "Initialize" {
            w236 = T4."Disabled and Grayed Out" ("Disabled")
            w237 = ""
            # "Initialize - Any operation that needs to be done before the module can receive messages. Synchronize Caller Events.vi will inform Start Module.vi that the module has launched and is ready to receive messages. Module Did Init.vi will broadcast that the module initialized."
            n140 = call "Synchronize Caller Events.vi"("error in"=w257, "Singleton Module Admin in"=w247) -> ("error out"=w256:errorcluster, "Singleton Module Admin out"=w242:refnum<class "Delacor_lib_QMH_Module Admin.lvclass">)  [unwired: 8 in]
            n141 = property on="Property Node" class="Module Admin"(reference=w242) -> ("Accessors:External Launch"=w251:bool)  [unwired: 1 in, 2 out]
            n142 = Select(t=T9."Hidden" ("State"), s=w251, f=T9."Standard" ("State")) -> (s? t:f=w248:T9)
            n143 = call "Module Name--constant.vi"() -> ("Module Name"=w254:string)  [unwired: 11 in]
            n144 = control-ref of="This VI"() -> (w239:refnum<vi>)
            n145 = property on="Property Node" class="VI"("Front Panel.Title"=w254) -> (reference out=w253:refnum<vi>, error out=w259:errorcluster)  [unwired: 2 in]
            n146 = invoke class="VI" method="Default Vals.Reinit All"(reference=w239, error in=w256) -> (error out=w240:errorcluster)  [unwired: 1 in, 2 out]
            n147 = Bundle By Name(cluster=w246, "Buffer"=w237, "Shift Status"=FALSE ("Uppercase Status")) -> (w245:T3)
            n148 = invoke on="Invoke Node" class="VI" method="FP.Open"(reference=w253, error in=w259, "State"=w248) -> (reference out=w252:refnum<vi>, error out=w258:errorcluster)  [unwired: 2 in, 3 out]
            n149 = invoke on="Invoke Node" class="VI" method="FP.Center"(reference=w252, error in=w258) -> ()  [unwired: 1 in, 3 out]
            n150 = property on="Pane" class="Pane"("Origin"=T8 {"Horizontal"=0, "Vertical"=0}) -> ()  [unwired: 2 in, 2 out]
            n151 = property on="Send" class="Bool"("DisabledEnum"=w236) -> ()  [unwired: 2 in, 2 out]
            n152 = property on="Buffer" class="Str"("DisabledEnum"=w236) -> ()  [unwired: 2 in, 2 out]
            n153 = call "Module Name--constant.vi"() -> ("Module Name"=w243:string)  [unwired: 11 in]
            n154 = call "Module Did Init.vi"("error in"=w240, "Initialized?"=TRUE, "Origin"=w243) -> ("error out"=w255:errorcluster)  [unwired: 8 in]
            "Status" <- w237
          }
          frame "---Module Specific---" {
            # "Separator -- The following cases handle messages specific to this Module."
          }
          frame "Get VI Refnum" {
            # "Return the module's VI refrum. This is usually used for inserting into a subpanel."
            n155 = Variant To Data(error in=w275, type=T7 {"Wait Notifier"=refnum, "wait for reply"=FALSE} ("Get VI Refnum Argument"), Variant=w271) -> (data=w269:T7, error out=w272:errorcluster)
            n156 = Unbundle By Name(w269) -> ("Wait Notifier"=w268:refnum<notifier>, "wait for reply"=w267:bool)
            n157 = control-ref of="This VI"() -> (w263:refnum<vi>)
            n158 = Bundle By Name(cluster=T10 {"VI Refnum"=refnum, "error"={"status"=FALSE, "code"=0, "source"=""}} ("Get VI Refnum (Reply Payload)"), "VI Refnum"=w263) -> (w266:T10)
            n159 = Merge Errors(w272) -> (w264:errorcluster)
            n160 = case "DQMH_FIRE_NOTIFIER" shown="True" w267 {
              tunnel: w268 -> [_ w277]
              tunnel: w266 -> [_ w276]
              frame False {
              }
              frame True {
                n161 = Send Notification(notification=w276, notifier=w277) -> ()  [unwired: 1 in, 2 out]
              }
            }
          }
          frame "---Copy This Frame---" {
            # "Duplicate this frame when creating new messages.  Change this comment in the duplicated frame to describe this message."
            n162 = Merge Errors(w281) -> (w280:errorcluster)
          }
          frame "Clear Buffer" {
            w282 = ""
            # "Set the buffer and buffer indicator to empty string constant."
            n163 = Bundle By Name(cluster=w284, "Buffer"=w282) -> (w283:T3)
          }
          frame "Broadcast Buffer" {
            # "The send character broadcast can pull\ndouble duty here as it sends a string. \nA string is a string is a string."
            # "Send the contents of the buffer to any listening module or VI."
            n164 = Unbundle By Name(w287) -> ("Buffer"=w286:string)
            n165 = call "Send Character.vi"("error in"=w290, "Character to send"=w286) -> ("error out"=w288:errorcluster)  [unwired: 9 in]
          }
          frame "Backspace" {
            n166 = in-place {
              in-place-border: [w295] -> w291
              # "Remove the last value from\nthe string."
              n167 = in-place-cluster #1(w293) -> ("Buffer"=w297:string)
              n168 = String Length(string=w297) -> (length=w298:i32)
              n169 = Decrement(x=w298) -> (x-1=w296:i32)
              n170 = String Subset(string=w297, length (rest)=w296) -> (substring=w295:string)  [unwired: 1 in]
              n171 = in-place-cluster #1("Buffer"=w295) -> (w292:T3)
            }
          }
          frame "Broadcast Character" {
            # "Send the last typed character to any listening module or VI."
            n172 = Variant To Data(error in=w307, type="", Variant=w306) -> (data=w302:string, error out=w304:errorcluster)
            n173 = call "Send Character.vi"("error in"=w304, "Character to send"=w302) -> ("error out"=w303:errorcluster)  [unwired: 9 in]
            n174 = Unbundle By Name(w300) -> ("Shift Status"=w299:bool)
            n175 = case shown="True" w299 {
              frame False {
                # "No shift key detected. Do nothing. No need to change the keys."
              }
              frame True {
                # "Reset shift to lowercase.\nThis allows the first character\nto be uppercase, and reset\nto lowercase for the rest."
                n176 = property on="Shift Left" class="Bool (strict)"("Val(Sgnl)"=FALSE ("Value (Signaling)")) -> ()  [unwired: 2 in, 2 out]
              }
            }
          }
          frame "Populate Buffer" {
            # "Update the buffer typedef and the buffer indicator."
            n177 = Variant To Data(error in=w317, type="", Variant=w315) -> (data=w312:string, error out=w316:errorcluster)
            n178 = in-place {
              in-place-border: w312 -> [w320]
              in-place-border: [w319] -> w309
              n179 = in-place-cluster #2(w313) -> ("Buffer"=w321:string)
              n180 = Concatenate Strings(w321, w320) -> (w319:string)
              n181 = in-place-cluster #2("Buffer"=w319) -> (w311:T3)
            }
            n182 = Unbundle By Name(w311) -> ("Shift Status"=w310:bool)
            n183 = case shown="True" w310 {
              frame False {
                # "No shift key detected. Do nothing. No need to change the keys."
              }
              frame True {
                # "Reset shift to lowercase.\nThis allows the first character\nto be uppercase, and reset\nto lowercase for the rest."
                n184 = property on="Shift Left" class="Bool (strict)"("Val(Sgnl)"=FALSE ("Value (Signaling)")) -> ()  [unwired: 2 in, 2 out]
              }
            }
          }
          frame "Capitalize Keys" {
            # "Convert keys to uppercase or lowercase."
            n185 = Variant To Data(error in=w329, type=enum16{"Uppercase", "Lowercase"}."Lowercase" ("Upper / Lower Case"), Variant=w325) -> (data=w323:enum16{"Uppercase", "Lowercase"}, error out=w326:errorcluster)
            n186 = call "Shift Keys.vi"("Upper / Lower Case"=w323, "Button Refs"=w327) -> ()  [unwired: 10 in]
          }
          frame "Shift Keys" {
            # "Convert keys back and forth form lowercase to uppercase."
            n187 = Variant To Data(error in=w340, type=enum16{"Uppercase", "Lowercase"}."Lowercase" ("Upper / Lower Case"), Variant=w336) -> (data=w334:enum16{"Uppercase", "Lowercase"}, error out=w337:errorcluster)
            n188 = call "Shift Keys.vi"("Upper / Lower Case"=w334, "Button Refs"=w338) -> ()  [unwired: 10 in]
            n189 = Equal?(x=w334, y=enum16{"Uppercase", "Lowercase"}."Uppercase" ("Upper / Lower Case")) -> (x = y?=w331:bool)
            n190 = Bundle By Name(cluster=w339, "Shift Status"=w331) -> (w332:T3)
          }
          frame "---Exit and Error Handling---" {
            # "Separator - The following cases handle errors and exit messages."
          }
          frame "Simulate MHL Error" {
            # "#DQMH_HowTo The 'Simulate MHL Error' button  illustrates how the MHL handles errors. This event is instructional in nature and can be removed."
            # "Simulate an error occurring at the MHL"
            n191 = call "Module Name--constant.vi"() -> ("Module Name"=w346:string)  [unwired: 11 in]
            n192 = Format Into String(format string="Simulated error originating at Message Handling Loop in %s", w346) -> (resulting string=w347:string)  [unwired: 2 in, 1 out]
            n193 = call <vilib>:"Error Cluster From Error Code.vi"("show call chain? (False)"=TRUE, "error message (\"\")"=w347, "error code (0)"=5001) -> ("error out"=w351:errorcluster)  [unwired: 6 in]
            n194 = Merge Errors(w353, w351) -> (w352:errorcluster)
          }
          frame "Error" {
            # "#DQMH_CodeRecommended - If the module is running in standalone mode (External Launch = FALSE), this code will pop up an error dialog and call the 'Exit' message if an error occurs. Add more fine-grained error management here."
            # "Error - Check the error message data and respond accordingly. This message is sent by the \"Error Handler\" VIs at the end of each loop in this application."
            n195 = property on="Property Node" class="Module Admin"(reference=w357) -> ("Accessors:External Launch"=w356:bool)  [unwired: 1 in, 2 out]
            n196 = Variant To Data(error in=w365, type=errorcluster {"status"=FALSE, "code"=0, "source"=""} ("error constant"), Variant=w359) -> (data=w355:errorcluster, error out=w363:errorcluster)
            n197 = local write "error out"(w355) -> ()
            n198 = call "Error Reported.vi"("Error"=w355) -> ()  [unwired: 10 in, 1 out]
            n199 = case shown="False" w356 {
              tunnel: [w370 _] -> w362
              tunnel: w358 -> [w368 _]
              tunnel: w355 -> [w369 _]
              frame False {
                n200 = disable-structure shown="Default" {
                  disable-tunnel: w369 -> [w371 _]
                  frame condition #0 (active) {
                    # "If the module is running standalone, then pop up an error dialog and call the \"Exit\" message."
                    n201 = call <vilib>:"Simple Error Handler.vi"("error in (no error)"=w371) -> ()  [unwired: 4 in, 5 out]
                  }
                  frame condition #1 {
                    # "To prevent the Simple Error Handler VI from being loaded (e.g. when deploying to a Real-Time target), add the Conditional Disable Symbol \"DQMH_Disable_SEH\" to your project and set it to TRUE."
                  }
                }
                n202 = call-poly <vilib>:"Delacor_lib_QMH_Enqueue Message (poly).vi"("Priority Message? (F)"=TRUE, "Message"="Exit", "Message Queue in"=w368) -> ("error out"=w370:errorcluster)  [unwired: 7 in, 1 out]
              }
              frame True {
                # "If the module was launched externally, calling the Error Reported broadcast VI is the only action performed by the \"Error\" message. The module's caller can then process the error appropriately."
              }
            }
            n203 = Merge Errors(w363, w362) -> (w361:errorcluster)
          }
          frame "Exit" {
            w377 = 91  # 91: not all Exit messages will have an argument
            w379 = TRUE  # Stop the VI
            # "Release the message queue reference"
            # "Exit - Exit the application."
            n204 = Variant To Data(error in=w387, type=T6 {"Origin"="", "Exit via Stop Module Req?"=FALSE, "Wait for Module to stop?"=FALSE} ("Stop Argument"), Variant=w378) -> (data=w375:T6, error out=w384:errorcluster)
            n205 = call <vilib>:"Clear Errors.vi"("error in (no error)"=w384, "specific error code to clear (0: all)"=w377) -> ("error out"=w386:errorcluster)  [unwired: 4 in, 1 out]
            n206 = control-ref of="This VI"() -> (w374:refnum<vi>)
            n207 = call-dynamic "Delacor_lib_QMH_Release Message Queue.vi"("error in"=w386, "Message Queue"=w381) -> ("error out"=w385:errorcluster)  [unwired: 9 in]
            n208 = call "Handle Exit.vi"("Stop Argument"=w375, "Admin in"=w373, "VI reference"=w374) -> ("error out"=w383:errorcluster)  [unwired: 7 in, 1 out]
            n209 = Merge Errors(w385, w383) -> (w382:errorcluster)
            n210 = call "Error Reported.vi"("Error"=w382) -> ()  [unwired: 10 in, 1 out]
          }
          frame Default {
            # "'Default' case only runs if there is a message that isn't defined in any of the other cases.  Output a programming error."
            n211 = call "Module Name--constant.vi"() -> ("Module Name"=w393:string)  [unwired: 11 in]
            n212 = Format Into String(format string="The invalid message string \"%s\" was received in the Message Handling Loop for module \"%s\".", w394, w393) -> (resulting string=w389:string)  [unwired: 2 in, 1 out]
            n213 = call <vilib>:"Error Cluster From Error Code.vi"("show call chain? (False)"=TRUE, "error message (\"\")"=w389, "error code (0)"=1) -> ("error out"=w396:errorcluster)  [unwired: 6 in]
            n214 = Merge Errors(w397, w396) -> (w398:errorcluster)
          }
        }
        "Buffer" <- w222
        n215 = call-dynamic "Delacor_lib_QMH_Error Handler - Message Handling Loop.vi"("error in"=w226, "Message Queue in"=w225) -> ("dup error in"=w227:errorcluster)  [unwired: 8 in, 1 out]
      }
    }
    frame Error {
      # "Synchronize Caller Events.vi will inform Start Module.vi that the module has launched and will let the code calling Start Module.vi register for broadcasts and would permit the caller receive the broadcast that an error occurred at launch time."
      n216 = call-dynamic "Delacor_lib_QMH_Release Message Queue.vi"("error in"=w406, "Message Queue"=w399) -> ("error out"=w405:errorcluster)  [unwired: 9 in]
      n217 = call "Synchronize Caller Events.vi"("Singleton Module Admin in"=w400) -> ("error out"=w407:errorcluster)  [unwired: 9 in, 1 out]
      n218 = call "Module Name--constant.vi"() -> ("Module Name"=w403:string)  [unwired: 11 in]
      n219 = Format Into String(format string="An error occurred during initialization. %s is no longer running.", w403) -> (resulting string=w401:string)  [unwired: 2 in, 1 out]
      n220 = Merge Errors(w405, w407) -> (w408:errorcluster)
      n221 = call "Error Reported.vi"("Additional Information"=w401, "Error"=w408) -> ()  [unwired: 9 in, 1 out]
    }
  }
  n222 = Merge Errors(w62, w65) -> (w61:errorcluster)
  n223 = call "Close Module.vi"("error in"=w61, "Module Admin in"=w56) -> ("error out"=w63:errorcluster, "External Launch"=w49:bool, "Module Admin out"=w50:refnum<class "Delacor_lib_QMH_Module Admin.lvclass">)  [unwired: 7 in]
  n224 = Unregister For Events(event registration refnum=w55, error in=w63) -> (error out=w60:errorcluster)
  "error out" <- w60
  n225 = case "External Launch?" shown="False" w49 {
    tunnel: w60 -> [_ w409]
    frame False {
    }
    frame True {
      n226 = case shown="No Error" w409 {
        frame No Error {
          n227 = disable-structure shown="Disabled" {
            frame Disabled {
              n228 = invoke on="Invoke Node" class="VI" method="FP.Close"() -> ()  [unwired: 3 in, 3 out]
            }
            frame Enabled {
            }
          }
        }
        frame Error {
          n229 = disable-structure shown="Default" {
            frame condition #0 (active) {
              n230 = invoke class="VI" method="FP.Open"("Activate"=TRUE ("Activate?")) -> ()  [unwired: 4 in, 5 out]
            }
            frame condition #1 {
              # "Don't show panel on error if running inside a built EXE."
            }
          }
        }
      }
    }
  }
  n231 = local write "Module Admin"(w50) -> ()
